vi "AR_Envelope_Generation_subVI.vi"(9 "Release in":i32, 10 "Attack  in":i32, 11 "Number of Samples in":dbl) -> (0 "Envelope XY Graph out":cluster{dbl[], dbl[]}, 3 "Envelope Array out":dbl[](array[numeric]))   [LabVIEW 2024]
doc: "This SubVI takes the number of samples, and ADSR variables. From this info, subVI creates an array of amplitude (MIN = 0, MAX = 1) for every sample acording to the ADSR variables.\nSubVI also creates a XY graph of created envelope.\n\nIN: Number of Samples; Attack; Release;\nOUT: Envelope Array, Envelope XY Graph;"
panel:
  out "b":dbl
  in  "Sustain in":i32
  out "XY Graph":cluster{dbl[], dbl[]}(graph)
  in  "Decay in":i32
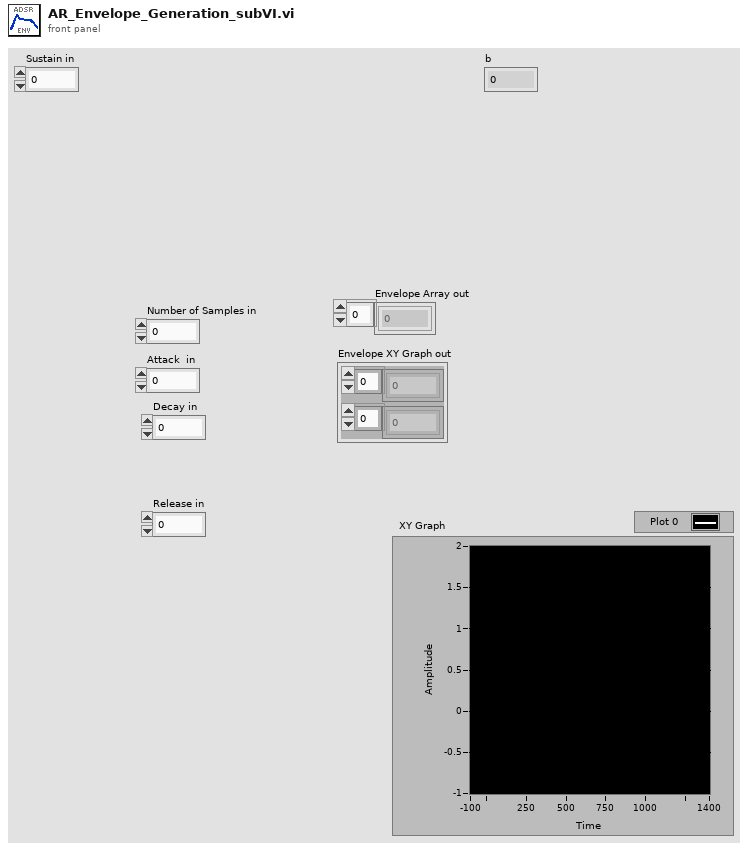
[diagram p1: front panel]
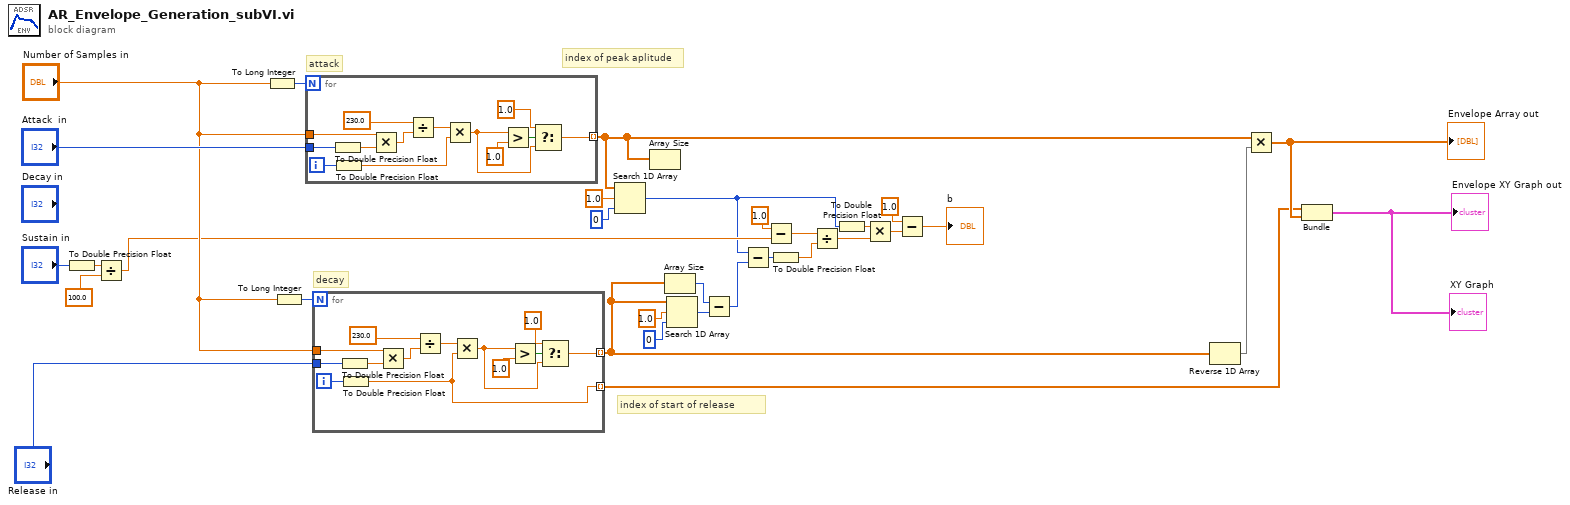
[diagram p0: block diagram]
diagram:
  # "index of start of release"
  # "index of peak aplitude"
  # "attack"
  # "decay"
  n1 = To Double Precision Float(number="Sustain in") -> (double precision float=w13:dbl)
  n2 = Divide(x=w13, y=100.0) -> (x/y=w11:dbl)
  n3 = To Long Integer(number="Number of Samples in") -> (32bit integer=w25:i32)
  n4 = To Long Integer(number="Number of Samples in") -> (32bit integer=w26:i32)
  n5 = for {
    N: w25 -> [_]
    tunnel: [w36] -> w21 mode=indexing
    tunnel: "Number of Samples in" -> [w35]
    tunnel: "Attack  in" -> [w33]
    i -> [w45]
    n6 = To Double Precision Float(number=w33) -> (double precision float=w34:dbl)
    n7 = To Double Precision Float(number=w45) -> (double precision float=w38:dbl)
    n8 = Multiply(x=w35, y=w34) -> (x*y=w40:dbl)
    n9 = Divide(x=230.0, y=w40) -> (x/y=w39:dbl)
    n10 = Multiply(x=w39, y=w38) -> (x*y=w37:dbl)
    n11 = Greater?(x=w37, y=1.0) -> (0:w44:bool)
    n12 = Select(t=1.0, s=w44, f=w37) -> (s? t:f=w36:dbl)
  }
  n13 = for {
    N: w26 -> [_]
    tunnel: [w52] -> w18 mode=indexing
    tunnel: "Number of Samples in" -> [w51]
    tunnel: [w49] -> w29 mode=indexing
    tunnel: "Release in" -> [w48]
    i -> [w58]
    n14 = To Double Precision Float(number=w48) -> (double precision float=w50:dbl)
    n15 = To Double Precision Float(number=w58) -> (double precision float=w49:dbl)
    n16 = Multiply(x=w51, y=w50) -> (x*y=w55:dbl)
    n17 = Divide(x=230.0, y=w55) -> (x/y=w54:dbl)
    n18 = Multiply(x=w54, y=w49) -> (x*y=w53:dbl)
    n19 = Greater?(x=w53, y=1.0) -> (0:w57:bool)
    n20 = Select(t=1.0, s=w57, f=w53) -> (s? t:f=w52:dbl)
  }
  n21 = Search 1D Array(1D array=w21, element=1.0, start index (0)=0) -> (index of element=w6:i32)
  n22 = Array Size(array=w21) -> ()  [unwired: 1 out]
  n23 = Array Size(array=w18) -> (size(s)=w16:i32)
  n24 = Search 1D Array(1D array=w18, element=1.0, start index (0)=0) -> (index of element=w17:i32)
  n25 = Subtract(x=w16, y=w17) -> (x-y=w9:i32)
  n26 = Subtract(x=w6, y=w9) -> (x-y=w8:i32)
  n27 = Subtract(x=1.0, y=w11) -> (x-y=w10:dbl)
  n28 = To Double Precision Float(number=w8) -> (double precision float=w7:dbl)
  n29 = Divide(x=w10, y=w7) -> (x/y=w5:dbl)
  n30 = To Double Precision Float(number=w6) -> (double precision float=w4:dbl)
  n31 = Multiply(x=w4, y=w5) -> (x*y=w2:dbl)
  n32 = Subtract(x=1.0, y=w2) -> (x-y=→"b":dbl)
  n33 = Reverse 1D Array(array=w18) -> (reversed array=w28:dbl[])
  n34 = Multiply(x=w21, y=w28) -> (x*y=w32:dbl[])
  "Envelope Array out" <- w32
  n35 = Bundle(w29, w32) -> (→"Envelope XY Graph out" →"XY Graph":cluster{dbl[], dbl[]})  [unwired: 1 in]
